vi "Read Command.vi"(8 "error in (no error)":errorcluster, 9 "timeout (100 ms)":i32=100, 11 "VeriStand Comm in":refnum<class "VeriStand Comm.lvclass">) -> (0 "error out":errorcluster, 1 "message value":string, 2 "message name":string, 3 "VeriStand Comm out":refnum<class "VeriStand Comm.lvclass">, 4 "ResponseInfo":T1, 5 "timed out?":bool)   [LabVIEW 2018, in "NI VeriStand Addon Network Comm.lvlib" / "VeriStand Comm.lvclass"]
uses:
  VeriStand Comm.lvclass
  _Types/Response Information.ctl
  VeriStand Comm.lvclass/VeriStand Comm.ctl
  <vilib>/NI/AMC/Read Termination Message.vi
  <vilib>/NI/Tools/Keyed Array/Map String.vi
  <vilib>/NI/AMC/Create Single Message.vi
  <vilib>/NI/Tools/String/Get Case Matching.vi
  Shared/Comm Constants.vi
  <vilib>/NI/AMC/Globals.vi
  <vilib>/NI/AMC/AMC.lvlib
  <vilib>/NI/Tools/Keyed Array/Tools_KeyedArray.lvlib
  Shared/NI VeriStand Addon Network Comm Shared.lvlib
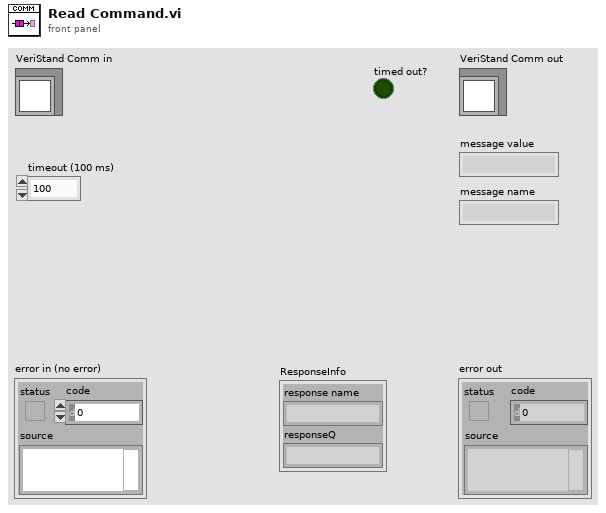
[diagram p1: front panel]
types:
  T1 = typedef "NI VeriStand Addon Network Comm.lvlib/VeriStand Comm.lvclass/Response Information.ctl" = cluster{"response name":string, "responseQ":string}
  T2 = typedef "AMC.lvlib/Message Queue.ctl" = refnum<queue>
  T3 = typedef "AMC.lvlib/Message.ctl" = cluster{"name":string, "value":string, "attributes":T4, "receiver host":string, "receiver process":string, "source host":string, "source process":string, "priority message":bool, "acknowledge message":bool}
  T4 = typedef "Tools_KeyedArray.lvlib/KeyedArray.ctl" = cluster{"keys":string[], "values":string[]}
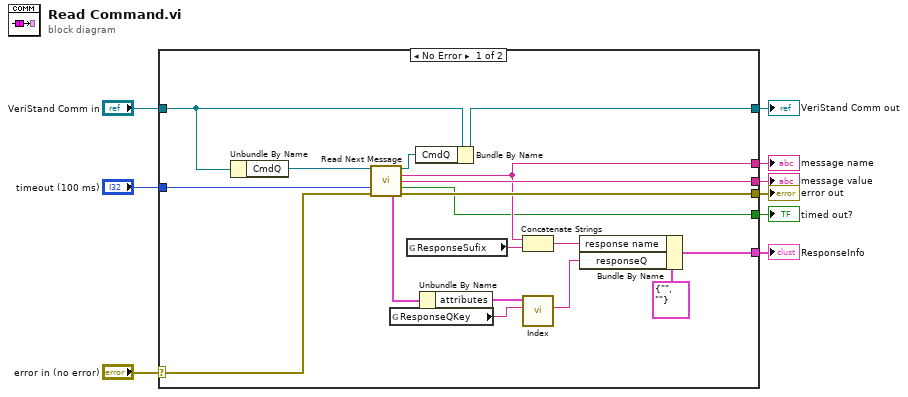
[diagram p0: block diagram]
diagram:
  n1 = case shown="No Error" "error in (no error)" {
    selector: "error in (no error)" -> [w23 w29]
    tunnel: [w22 w29] -> w8
    tunnel: [w11 w28] -> w6
    tunnel: "VeriStand Comm in" -> [w12 w28]
    tunnel: [w20 _] -> w5
    tunnel: [w19 _] -> w4
    tunnel: "timeout (100 ms)" -> [w18 _]
    tunnel: [w14 _] -> w2
    tunnel: [w10 _] -> w1
    frame No Error {
      n2 = Unbundle By Name(w12) -> ("CmdQ"=w24:T2)
      n3 = call <vilib>:"Read Next Message.vi"("message queue in"=w24, "timeout (1 ms)"=w18, "error in"=w23) -> ("message queue out"=w13:T2, "message name"=w19:string, "message value"=w20:string, "timed out?"=w10:bool, "message"=w25:T3, "error out"=w22:errorcluster)  [unwired: 5 in, 2 out]
      n4 = global read "Comm Constants.vi" "ResponseQKey"() -> (w27:string)
      n5 = global read "Comm Constants.vi" "ResponseSufix"() -> (w21:string)
      n6 = Bundle By Name(cluster=w12, "CmdQ"=w13) -> (w11:refnum<class "VeriStand Comm.lvclass">)
      n7 = Unbundle By Name(w25) -> ("attributes"=w26:T4)
      n8 = Concatenate Strings(w19, w21) -> (w17:string)
      n9 = call <vilib>:"Index.vi"("key"=w27, "array in"=w26) -> ("value"=w16:string)  [unwired: 3 in, 2 out]
      n10 = Bundle By Name(cluster=T1 {"response name"="", "responseQ"=""}, "response name"=w17, "responseQ"=w16) -> (w14:T1)
    }
    frame Error {
    }
  }
  "error out" <- w8
  "VeriStand Comm out" <- w6
  "message value" <- w5
  "message name" <- w4
  "ResponseInfo" <- w2
  "timed out?" <- w1
